vi "Protocol Read.vi"(8 "error in (no error)":errorcluster, 10 "bytes to read":i32, 11 "TCP in":refnum<class "TCP.lvclass">) -> (0 "error out":errorcluster, 1 "timed out?":bool, 2 "data":u8[](array[numeric]), 3 "TCP out":refnum<class "TCP.lvclass">)   [LabVIEW 2021, in "TCP.lvclass"]
doc: "Reads from the established TCP connection stored in the class."
uses:
  TCP.lvclass
  TCP.lvclass/TCP.ctl
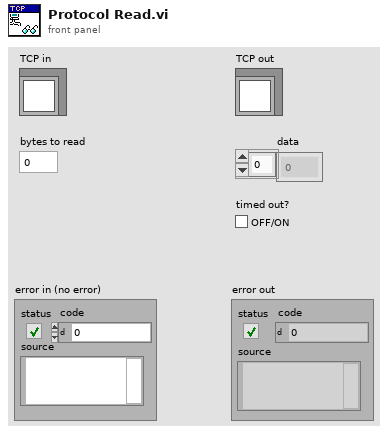
[diagram p1: front panel]
types:
  T1 = enum16{"Standard", "Buffered", "CRLF", "Immediate"}
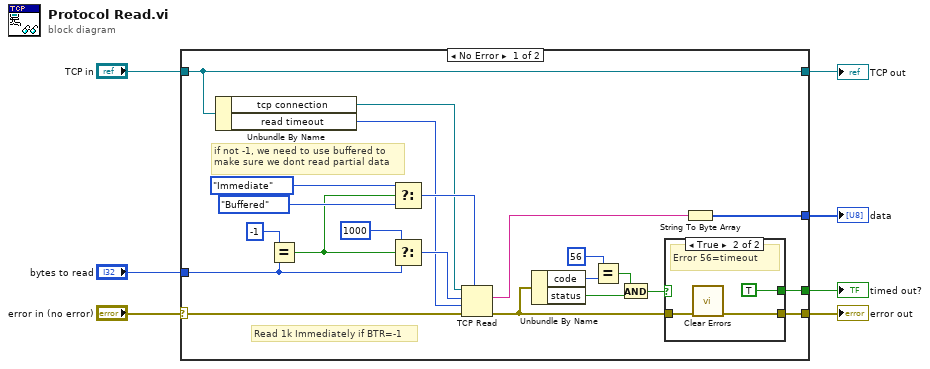
[diagram p0: block diagram]
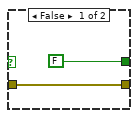
[diagram p2: hidden frame]
diagram:
  n1 = case shown="No Error" "error in (no error)" {
    selector: "error in (no error)" -> [w18 w36]
    tunnel: [w29 w36] -> w4
    tunnel: [w28 _] -> w5
    tunnel: "bytes to read" -> [w21 _]
    tunnel: [w17 _] -> w3
    tunnel: "TCP in" -> [w10 w35]
    tunnel: [w10 w35] -> w1
    frame No Error {
      # "Read 1k Immediately if BTR=-1"
      # "if not -1, we need to use buffered to\nmake sure we dont read partial data"
      n2 = Unbundle By Name(w10) -> ("tcp connection"=w9:refnum<k5>, "read timeout"=w8:i32)
      n3 = Equal?(x=-1, y=w21) -> (x = y?=w22:bool)
      n4 = Select(t=T1."Immediate" ("mode (standard)"), s=w22, f=T1."Buffered" ("mode (standard)")) -> (s? t:f=w23:T1)
      n5 = Select(t=1000, s=w22, f=w21) -> (s? t:f=w20:i32)
      n6 = TCP Read(connection ID=w9, bytes to read=w20, error in (no error)=w18, 7:w23, 9:w8) -> (data out=w27:string, error out=w11:errorcluster)  [unwired: 1 out]
      n7 = Unbundle By Name(w11) -> ("code"=w16:i32, "status"=w13:bool)
      n8 = Equal?(x=56, y=w16) -> (x = y?=w14:bool)
      n9 = And(x=w14, y=w13) -> (x .and. y?=w12:bool)
      n10 = case shown="True" w12 {
        tunnel: w11 -> [w31 w33]
        tunnel: [w31 w32] -> w29
        tunnel: [FALSE TRUE] -> w17
        frame False {
        }
        frame True {
          # "Error 56=timeout"
          n11 = call <vilib>:"Clear Errors.vi"("error in (no error)"=w33) -> ("error out"=w32:errorcluster)  [unwired: 5 in, 1 out]
        }
      }
      n12 = String To Byte Array(string=w27) -> (unsigned byte array=w28:u8[])
    }
    frame Error {
    }
  }
  "error out" <- w4
  "TCP out" <- w1
  "data" <- w5
  "timed out?" <- w3
